vi "Test Reshape to 1D Array.vi"() -> ()   [LabVIEW 2018]
panel:
  out "size(s)":i32
  out "time for reshape":dbl
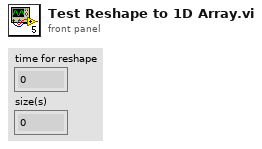
[diagram p1: front panel]
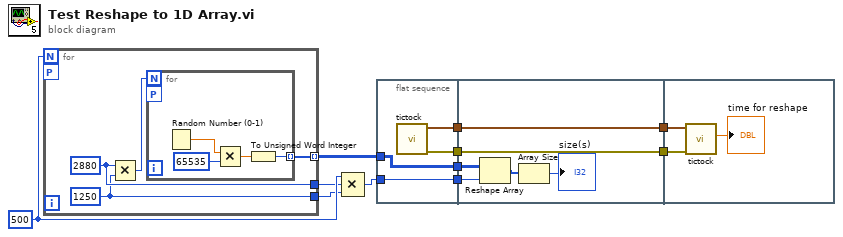
[diagram p0: block diagram]
diagram:
  w10 = 500
  n1 = for {
    N: w10 -> [_]
    tunnel: [w14] -> w11 mode=indexing
    tunnel: [w13] -> w9
    tunnel: [w12] -> w8
    workers-P: _ -> [_]
    w12 = 1250
    w13 = 2880
    n2 = Multiply(x=w13, y=w12) -> (x*y=w15:i32)
    n3 = for {
      N: w15 -> [_]
      tunnel: [w16] -> w14 mode=indexing
      workers-P: _ -> [_]
      n4 = Random Number (0-1)() -> (number: 0 to 1=w19:dbl)
      n5 = Multiply(x=w19, y=u16 65535) -> (x*y=w17:dbl)
      n6 = To Unsigned Word Integer(number=w17) -> (unsigned 16bit integer=w16:u16)
    }
  }
  n7 = Compound Arithmetic op=MULTIPLY(w10, w9, w8) -> (w7:i32)
  n8 = flat-sequence {
    tunnel: w7 -> [w22]
    tunnel: w11 -> [w23]
    tunnel: [w23] -> w6
    tunnel: [w22] -> w5
    tunnel: [w21] -> w3
    tunnel: [w20] -> w2
    tunnel: w6 -> [w29]
    tunnel: w5 -> [w28]
    tunnel: [w27] -> w4
    tunnel: w3 -> [w27]
    tunnel: w2 -> [w26]
    tunnel: [w26] -> w1
    tunnel: w4 -> [w32]
    tunnel: w1 -> [w31]
    frame #0 {
      n9 = call "tictock.vi"() -> ("error out"=w21:errorcluster, "seconds since 1Jan1904"=w20:timestamp)  [unwired: 9 in, 1 out]
    }
    frame #1 {
      n10 = Reshape Array(w29, w28) -> (w25:u16[])
      n11 = Array Size(array=w25) -> (size(s)=→"size(s)":i32)
    }
    frame #2 {
      n12 = call "tictock.vi"("error in (no error)"=w32, "seconds since 1Jan1904 2"=w31) -> ("Numeric"=→"time for reshape":dbl)  [unwired: 7 in, 2 out]
    }
  }
